vi "Experiment header-bundle and save.vi"(8 "error in (no error)":errorcluster, 10 "AOL_Globals":T1={"Imaging Protocol"=enum."AOL Z-Stack", "Number of POI"=0, "Number of Miniscans"=0, "Number of Trials"=0, "Number of Cycles "=0, "# Averaged Frames"=0, "Laser power (%)"=0, "Pockels (V)"=0.0, "Acquisition Length (sec)"=0.0, "Fill time (us)"=0.0, "POI Dwell time (us)"=0.0, "Miniscan Dwell time per pixel (us)"=0.0, "PMT 1"=0.0, "PMT 2"=0.0, "Back Apperture (mA)"=200.0, "Frame Size"=0, "Center Frequency"=0.0, "Field of View (um)"=175.0, "Field of View (norm)"=0.0, "DwellTime (us)"=0.0, "Ref Dwell Time (us)"=0.0, "Wavelength (nm)"=0.0, "Zoom"=0.0, "AOL Z"=0.0, "AOL Mode"=enum."Raster", "GridXY"=0.0, "GridZ"=0.0, "TriggerPeriod (sec)"=0.0, "Number of Pixels in Miniscan"=0, "Experiment folder path"=path "", "X centre"=0.0, "Y centre"=0.0, "Angle (degrees)"=0.0, "Angle Xs (degrees)"=0.0, "Angle Ys (degrees)"=0.0, "Plane Mode"=0, "Threshold"=[], "Regenerate Chirps"=FALSE, "Rectangle ROI length (pixels)"=0, "Rectangle ROI height (pixels)"=0, "AOD fill"=4900, "StartupDelay"=0, "Samples Wait after Trigger"=5080, "Slip Cycle"=600000, "Add Cycle"=TRUE, "Functional Mode"=enum."Point", "Z Start"=0.0, "Z Stop"=0.0, "# Planes"=0, "Total Pixels"=0, "Variable Miniscan Pixels"=[], "Use Variable Length"=FALSE, "Use Variable Resolution"=FALSE, "Laser power (%) at Z Start"=0, "Laser power (%) at Z Stop"=0, "Ref Z Step"=0} {"Angle Ys (degrees)" format="%#.6g"; "Angle Xs (degrees)" format="%#.6g"; "Plane Mode" items=["XY Plane", "XZ Plane", "YZ Plane", "arbitraryplane"]; "Frame Size" items=["100X100"=100, "128X128"=128, "200X200"=200, "256X256"=256, "512X512"=512, "1024x1024"=1024, "2048x2048"=2048]; "Back Apperture (mA)" format="%#.6g"; "Pockels (V)" format="%#.6g"; "PMT 2" format="%#.6g"; "PMT 1" format="%#.6g"; "Angle (degrees)" format="%#.6g"; "POI Dwell time (us)" format="%#.6g"}, 11 "Experiment data folder path":path) -> (0 "error out":errorcluster)   [LabVIEW 2020]
uses:
  Typedefs/Controls/AOL_Globals.ctl
  Typedefs/Imaging Protocols enum.ctl
  Typedefs/Frame Size.ctl
  Typedefs/AOL modes.ctl
  Typedefs/Plane Mode.ctl
  Typedefs/Functional Mode.ctl
  Typedefs/Header file interface module functions enum.ctl
  Typedefs/Header file sections.ctl
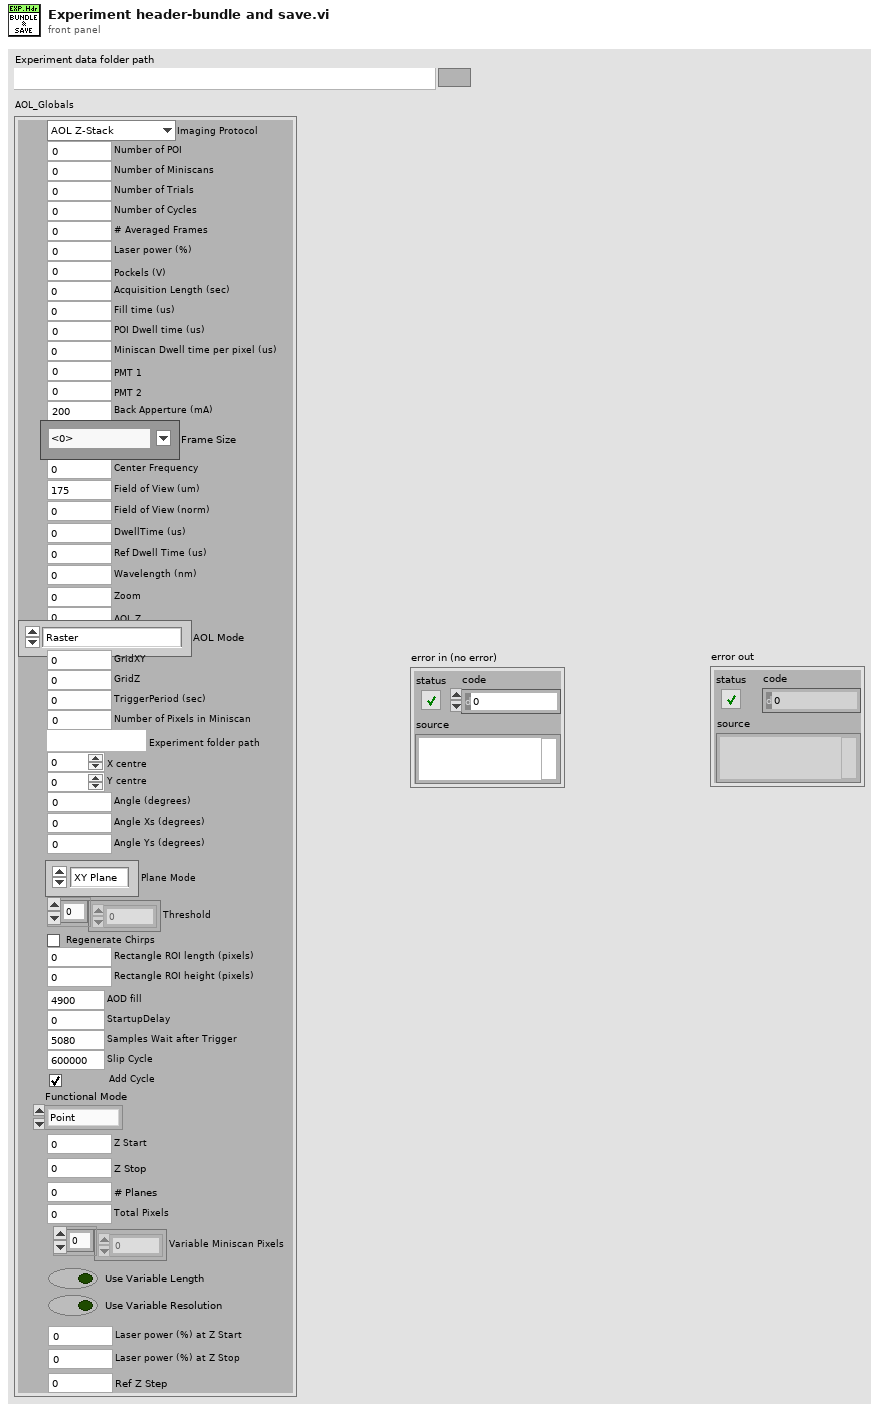
[diagram p1: front panel]
types:
  T1 = typedef "AOL_Globals.ctl" = cluster{"Imaging Protocol":T2, "Number of POI":u16, "Number of Miniscans":u16, "Number of Trials":u16, "Number of Cycles ":u64, "# Averaged Frames":u16, "Laser power (%)":u8, "Pockels (V)":dbl, "Acquisition Length (sec)":dbl, "Fill time (us)":dbl, "POI Dwell time (us)":dbl, "Miniscan Dwell time per pixel (us)":dbl, "PMT 1":dbl, "PMT 2":dbl, "Back Apperture (mA)":dbl, "Frame Size":T3, "Center Frequency":dbl, "Field of View (um)":dbl, "Field of View (norm)":dbl, "DwellTime (us)":dbl, "Ref Dwell Time (us)":dbl, "Wavelength (nm)":dbl, "Zoom":dbl, "AOL Z":dbl, "AOL Mode":T4, "GridXY":dbl, "GridZ":dbl, "TriggerPeriod (sec)":dbl, "Number of Pixels in Miniscan":u16, "Experiment folder path":path, "X centre":dbl, "Y centre":dbl, "Angle (degrees)":dbl, "Angle Xs (degrees)":dbl, "Angle Ys (degrees)":dbl, "Plane Mode":T5, "Threshold":u16[], "Regenerate Chirps":bool, "Rectangle ROI length (pixels)":u16, "Rectangle ROI height (pixels)":u16, "AOD fill":u16, "StartupDelay":i32, "Samples Wait after Trigger":u16, "Slip Cycle":u32, "Add Cycle":bool, "Functional Mode":T6, "Z Start":dbl, "Z Stop":dbl, "# Planes":i32, "Total Pixels":i32, "Variable Miniscan Pixels":u16[], "Use Variable Length":bool, "Use Variable Resolution":bool, "Laser power (%) at Z Start":u8, "Laser power (%) at Z Stop":u8, "Ref Z Step":i8}
  T2 = typedef "Imaging Protocols enum.ctl" = enum16{"AOL Z-Stack", "Motor Z Stack", "Parameter Sweep", "Functional Acquisition", "Single Plane Acquisition", "Volume Acquisition", "Live Imaging", "Live Plane Imaging", "Live Volume Imaging"}
  T3 = typedef "Frame Size.ctl" = u16
  T4 = typedef "AOL modes.ctl" = enum16{"Raster", "Structural", "Pointing", "Mini Scan", "Alignment"}
  T5 = typedef "Plane Mode.ctl" = u16
  T6 = typedef "Functional Mode.ctl" = enum16{"Point", "Line", "Patch", "Plane", "Volume"}
  T7 = typedef "Header file sections.ctl" = enum16{"ALL SECTIONS", "LOGIN", "GLOBAL PARAMETERS", "CALIBRATION DATA", "IMAGING MODES", "TIME SERIES", "MOTOR Z-STACK", "AOL Z-STACK", "FUNCTIONAL IMAGING", "VOLUME IMAGING", "MOVEMENT CORRECTION", "CALIBRATION", "STATISTICS", "BIOLOGY INFORMATION"}
  T8 = typedef "Header file interface module functions enum.ctl" = enum16{"Load experiment header file", "Save experiment header file", "Clear stored values", "Read stored values", "Update specific value in memory", "Update values in memory"}
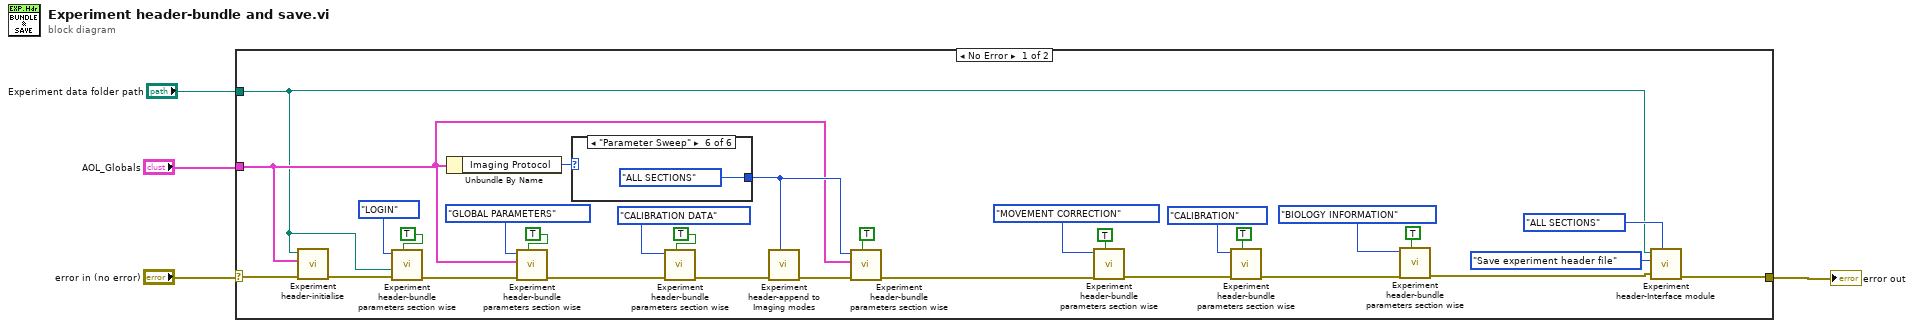
[diagram p0: block diagram]
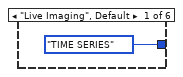
[diagram p2: hidden frame]
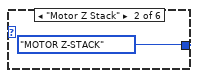
[diagram p3: hidden frame]
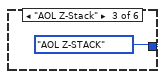
[diagram p4: hidden frame]
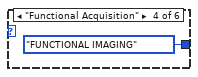
[diagram p5: hidden frame]
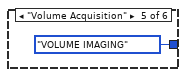
[diagram p6: hidden frame]
diagram:
  n1 = case shown="No Error" "error in (no error)" {
    selector: "error in (no error)" -> [w29 w41]
    tunnel: "AOL_Globals" -> [w22 _]
    tunnel: [w33 w41] -> w2
    tunnel: "Experiment data folder path" -> [w11 _]
    frame No Error {
      n2 = call "Experiment header-initialise.vi"("error in (no error)"=w29, "AOL_Globals"=w22, "Experiment data folder path"=w11) -> ("error out"=w26:errorcluster)  [unwired: 8 in]
      n3 = call "Experiment header-bundle parameters section wise.vi"("Update header\ninterface cluster ?"=TRUE ("Update header\ninterface cluster ?"), "error in (no error)"=w26, "Experiment data folder path"=w11, "Header file sections"=Header_file_sections."LOGIN") -> ("error out"=w21:errorcluster)  [unwired: 6 in, 1 out]
      n4 = Unbundle By Name(w22) -> ("Imaging Protocol"=w34:T2)
      n5 = call "Experiment header-bundle parameters section wise.vi"("Update header\ninterface cluster ?"=TRUE ("Update header\ninterface cluster ?"), "error in (no error)"=w21, "AOL_Globals"=w22, "Header file sections"=Header_file_sections."GLOBAL PARAMETERS") -> ("error out"=w10:errorcluster)  [unwired: 6 in, 1 out]
      n6 = case shown="\"Parameter Sweep\"" w34 {
        tunnel: [Header_file_sections."TIME SERIES" ("Header file sections") Header_file_sections."MOTOR Z-STACK" ("Header file sections") Header_file_sections."AOL Z-STACK" ("Header file sections") Header_file_sections."FUNCTIONAL IMAGING" ("Header file sections") Header_file_sections."VOLUME IMAGING" ("Header file sections") Header_file_sections."ALL SECTIONS" ("Header file sections")] -> w30
        frame "Live Imaging", Default {
        }
        frame "Motor Z Stack" {
        }
        frame "AOL Z-Stack" {
        }
        frame "Functional Acquisition" {
        }
        frame "Volume Acquisition" {
        }
        frame "Parameter Sweep" {
        }
      }
      n7 = call "Experiment header-bundle parameters section wise.vi"("Update header\ninterface cluster ?"=TRUE ("Update header\ninterface cluster ?"), "error in (no error)"=w10, "Header file sections"=Header_file_sections."CALIBRATION DATA") -> ("error out"=w9:errorcluster)  [unwired: 7 in, 1 out]
      n8 = call "Experiment header-append to Imaging modes.vi"("Header file sections"=w30, "error in (no error)"=w9) -> ("error out"=w31:errorcluster)  [unwired: 9 in]
      n9 = call "Experiment header-bundle parameters section wise.vi"("Update header\ninterface cluster ?"=TRUE ("Update header\ninterface cluster ?"), "error in (no error)"=w31, "AOL_Globals"=w22, "Header file sections"=w30) -> ("error out"=w5:errorcluster)  [unwired: 6 in, 1 out]
      n10 = call "Experiment header-bundle parameters section wise.vi"("Update header\ninterface cluster ?"=TRUE ("Update header\ninterface cluster ?"), "error in (no error)"=w5, "Header file sections"=Header_file_sections."MOVEMENT CORRECTION") -> ("error out"=w16:errorcluster)  [unwired: 7 in, 1 out]
      n11 = call "Experiment header-bundle parameters section wise.vi"("Update header\ninterface cluster ?"=TRUE ("Update header\ninterface cluster ?"), "error in (no error)"=w16, "Header file sections"=Header_file_sections."CALIBRATION") -> ("error out"=w13:errorcluster)  [unwired: 7 in, 1 out]
      n12 = call "Experiment header-bundle parameters section wise.vi"("Update header\ninterface cluster ?"=TRUE ("Update header\ninterface cluster ?"), "error in (no error)"=w13, "Header file sections"=Header_file_sections."BIOLOGY INFORMATION") -> ("error out"=w6:errorcluster)  [unwired: 7 in, 1 out]
      n13 = call "Experiment header-Interface module.vi"("Header file sections"=Header_file_sections."ALL SECTIONS", "error in (no error)"=w6, "Function"=Header_file_interface_module_functions_enum."Save experiment header file", "Experiment data folder path"=w11) -> ("error out"=w33:errorcluster)  [unwired: 6 in, 1 out]
    }
    frame Error {
    }
  }
  "error out" <- w2
